vi "Close IntClk Device.vi"(0 "Dig out task":refnum<k21>, 5 "Dig in task":refnum<k21>, 11 "error in":errorcluster) -> (15 "error out":errorcluster)   [LabVIEW 2016, in "SPIVI.lvlib"]
uses:
  SPIVI.lvlib
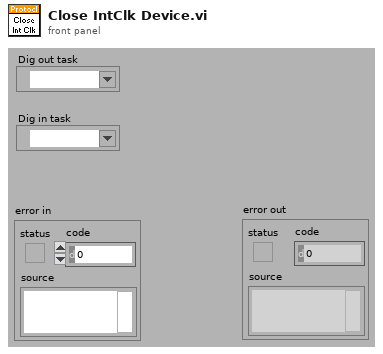
[diagram p1: front panel]
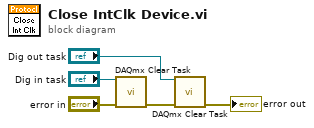
[diagram p0: block diagram]
diagram:
  n1 = call <vilib>:"DAQmx Clear Task.vi"("task in"="Dig in task", "error in"="error in") -> ("error out"=w5:errorcluster)  [unwired: 13 out]
  n2 = call <vilib>:"DAQmx Clear Task.vi"("task in"="Dig out task", "error in"=w5) -> ("error out"=→"error out":errorcluster)  [unwired: 13 out]
